vi "punias_save.vi"(8 "error in (no error)":errorcluster, 9 "datalog path (use dialog)":path, 11 "Cluster":T1) -> (0 "error out":errorcluster)   [LabVIEW 2013]
uses:
  <vilib>/regexp/Match Regular Expression.xnode
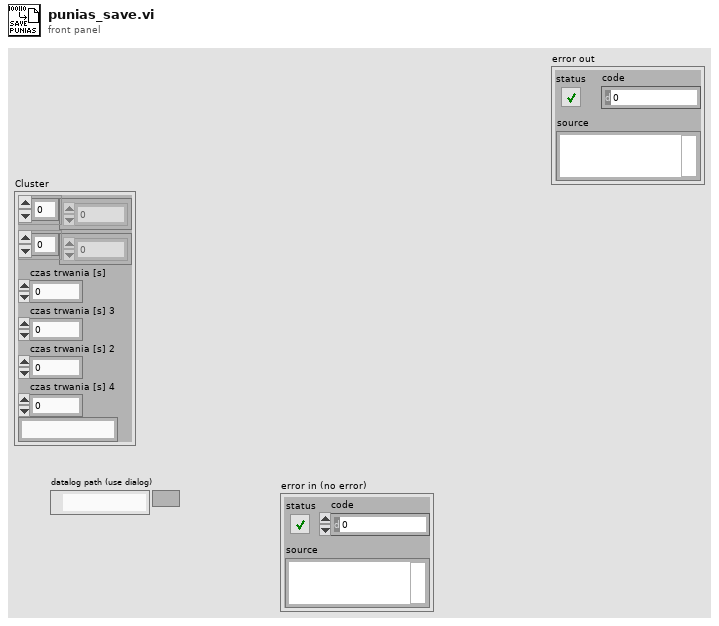
[diagram p1: front panel]
types:
  T1 = cluster{dbl[], dbl[], "czas trwania [s]":dbl, "czas trwania [s] 3":dbl, "czas trwania [s] 2":dbl, "czas trwania [s] 4":dbl, string}
  T2 = enum16{"open", "replace", "create", "open or create", "replace or create", "replace or create with confirmation"}
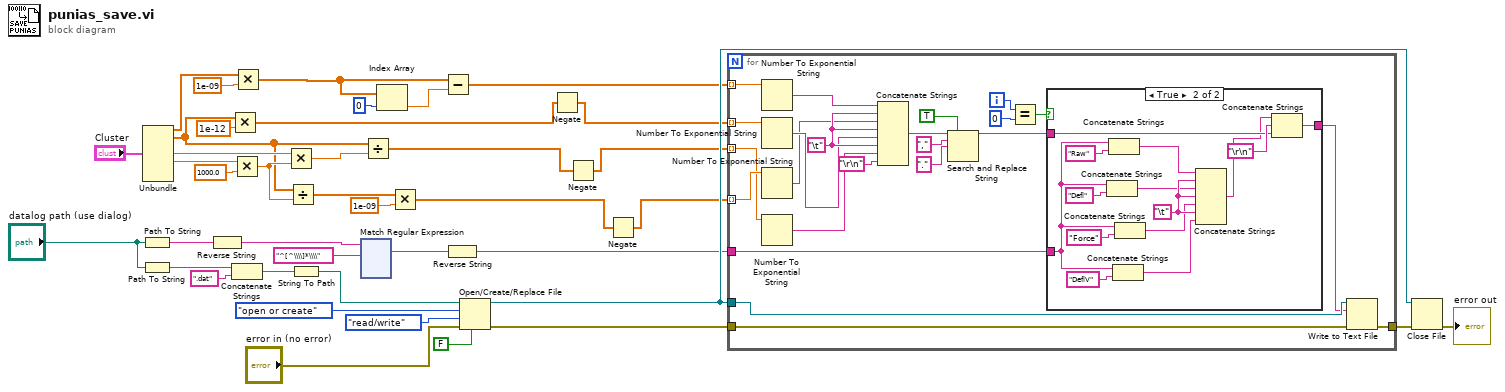
[diagram p0: block diagram]
diagram:
  n1 = Path To String(path="datalog path (use dialog)") -> (string=w25:string)
  n2 = Path To String(path="datalog path (use dialog)") -> (string=w35:string)
  n3 = Unbundle("Cluster") -> (w21:dbl[], w10:dbl[], "czas trwania [s] 3"=w15:dbl, "czas trwania [s] 2"=w12:dbl)  [unwired: 3 out]
  n4 = Reverse String(1:w25) -> (0:w27:string)
  n5 = Multiply(x=w10, y=1e-12) -> (x*y=w6:dbl[])
  n6 = Multiply(x=w12, y=1000.0) -> (x*y=w11:dbl)
  n7 = Concatenate Strings(w35, ".dat") -> (w34:string)
  n8 = Multiply(x=w21, y=1e-09) -> (x*y=w7:dbl[])
  n9 = Multiply(x=w15, y=w11) -> (x*y=w13:dbl)
  n10 = Divide(x=w10, y=w11) -> (x/y=w8:dbl[])
  n11 = String To Path(string=w34) -> (path=w33:path)
  n12 = xnode "Match Regular Expression"("input string"=w27, "regular expression"="^[^\\\\]*\\\\") -> ("whole match"=w22:string)  [unwired: 4 in, 4 out]
  n13 = Divide(x=w10, y=w13) -> (x/y=w4:dbl[])
  n14 = Index Array(array=w7, index=0) -> (element=w18:dbl)
  n15 = Multiply(x=w8, y=1e-09) -> (x*y=w2:dbl[])
  n16 = Subtract(x=w7, y=w18) -> (x-y=w17:dbl[])
  n17 = Reverse String(1:w22) -> (0:w23:string)
  n18 = Open/Create/Replace File(file path (use dialog)=w33, error in="error in (no error)", operation (0:open)=T2."open or create", access (0:read/write)=enum16{"read/write", "read-only", "write-only"}."read/write", disable buffering (F)=FALSE) -> (refnum out=w30:refnum<file>, error out=w29:errorcluster)  [unwired: 1 in, 1 out]
  n19 = Negate(x=w6) -> (-x=w5:dbl[])
  n20 = Negate(x=w4) -> (-x=w3:dbl[])
  n21 = Negate(x=w2) -> (-x=w1:dbl[])
  n22 = for {
    tunnel: w30 -> [w57]
    tunnel: w29 -> [w56]
    tunnel: w23 -> [w46]
    tunnel: [w45] -> w40
    tunnel: w17 -> [w44] mode=indexing
    tunnel: w5 -> [w43] mode=indexing
    tunnel: w1 -> [w42] mode=indexing
    tunnel: w3 -> [w41] mode=indexing
    i -> [w51]
    w63 = "\t"
    n23 = Number To Exponential String(number=w44) -> (E-format string=w61:string)  [unwired: 3 in]
    n24 = Number To Exponential String(number=w43) -> (E-format string=w60:string)  [unwired: 3 in]
    n25 = Number To Exponential String(number=w42) -> (E-format string=w59:string)  [unwired: 3 in]
    n26 = Number To Exponential String(number=w41) -> (E-format string=w58:string)  [unwired: 3 in]
    n27 = Concatenate Strings(w61, w63, w59, w63, w60, w63, w58, "\r\n") -> (w48:string)
    n28 = Search and Replace String(replace all?=TRUE ("replace all? (F)"), input string=w48, search string=",", replace string="." ("replace string (\"\")")) -> (result string=w49:string)  [unwired: 4 in, 3 out]
    n29 = Equal?(x=w51, y=0) -> (x = y?=w50:bool)
    n30 = case shown="True" w50 {
      tunnel: [w64 w77] -> w47
      tunnel: w49 -> [w64 w76]
      tunnel: w46 -> [_ w68]
      frame False {
      }
      frame True {
        w75 = "\t"
        n31 = Concatenate Strings(w68, "Defl" ("string")) -> (w65:string)
        n32 = Concatenate Strings(w68, "Raw" ("string")) -> (w72:string)
        n33 = Concatenate Strings(w68, "DeflV" ("string")) -> (w67:string)
        n34 = Concatenate Strings(w68, "Force" ("string")) -> (w66:string)
        n35 = Concatenate Strings(w72, w75, w65, w75, w66, w75, w67) -> (w74:string)
        n36 = Concatenate Strings(w74, "\r\n", w76) -> (w77:string)
      }
    }
    n37 = Write to Text File(file (use dialog)=w57, text=w47, error in=w56) -> (error out=w45:errorcluster)  [unwired: 1 in, 2 out]
  }
  n38 = Close File(refnum=w30, error in=w40) -> (error out=→"error out":errorcluster)  [unwired: 1 out]
